vi "Generate Shipping List.vi"(8 "error in (no error)":errorcluster, 10 "Shipping ID":i32, 11 "Delivery in":refnum<class "Delivery.lvclass">) -> (0 "error out":errorcluster, 3 "Delivery out":refnum<class "Delivery.lvclass">)   [LabVIEW 2019, in "Delivery.lvclass"]
uses:
  Delivery.lvclass
  Delivery.lvclass/Delivery.ctl
panel:
  out "Price:":string
  out "Estimated Delivery Time:":string
  out "Transport Company:":string
  out "Parcel Delivery Address":string
  out "Parcel Pickup Address":string
  out "Shipping List ID:":string
  out "Recipient:":string
  in  "Stop":bool
  out "Sender:":string
  # "Shipping List"
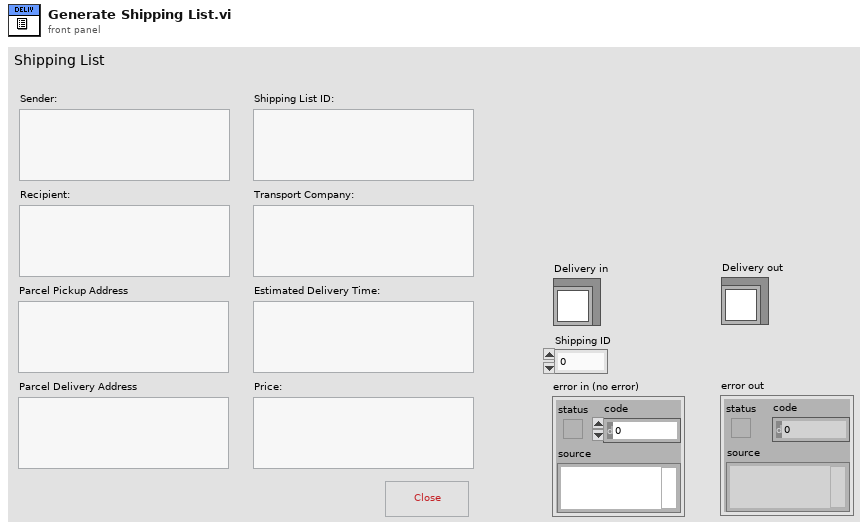
[diagram p1: front panel]
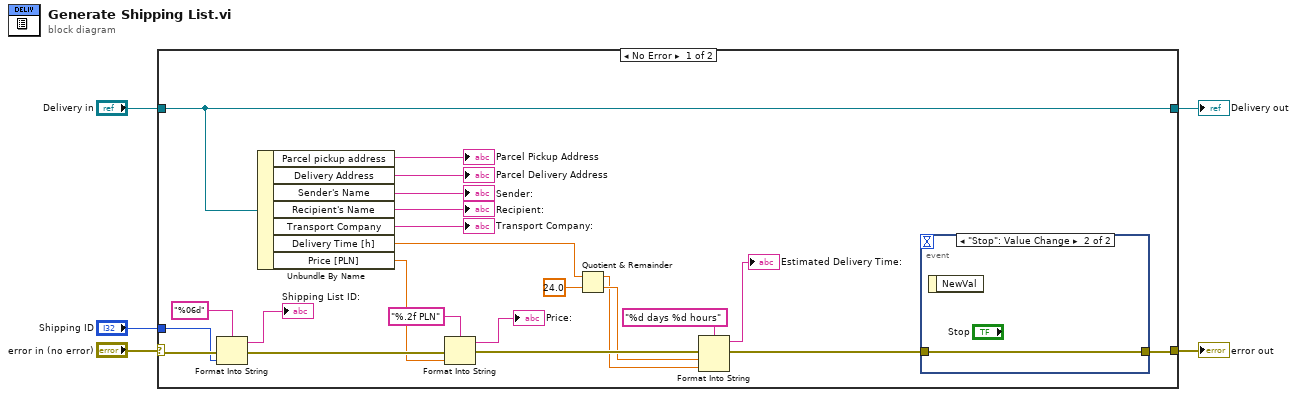
[diagram p0: block diagram]
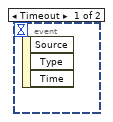
[diagram p2: hidden frame]
diagram:
  n1 = case shown="No Error" "error in (no error)" {
    selector: "error in (no error)" -> [w22 w31]
    tunnel: [w6 w31] -> w4
    tunnel: [w28 w30] -> w2
    tunnel: "Delivery in" -> [w28 w30]
    tunnel: "Shipping ID" -> [w20 _]
    frame No Error {
      n2 = Format Into String(format string="%06d", error in=w22, w20) -> (resulting string=→"Shipping List ID:":string, error out=w18:errorcluster)  [unwired: 1 in]
      n3 = Unbundle By Name(w28) -> ("Parcel pickup address"=→"Parcel Pickup Address":string, "Delivery Address"=→"Parcel Delivery Address":string, "Sender's Name"=→"Sender:":string, "Recipient's Name"=→"Recipient:":string, "Transport Company"=→"Transport Company:":string, "Delivery Time [h]"=w14:dbl, "Price [PLN]"=w17:dbl)
      n4 = Format Into String(format string="%.2f PLN", error in=w18, w17) -> (resulting string=→"Price:":string, error out=w12:errorcluster)  [unwired: 1 in]
      n5 = Quotient & Remainder(x=w14, y=24.0) -> (x-y*floor(x/y)=w9:dbl, floor(x/y)=w10:dbl)
      n6 = Format Into String(format string="%d days %d hours", error in=w12, w10, w9) -> (resulting string=→"Estimated Delivery Time:":string, error out=w7:errorcluster)  [unwired: 1 in]
      n7 = event shown="[1] \"Stop\": Value Change" {
        selector: _ -> [_ _]
        dyn-events: _ -> [_ _]
        timeout: _ -> [_ _]
        tunnel: w7 -> [_ w29]
        tunnel: [_ w29] -> w6
        event Timeout {
          n8 = event-data() -> ()  [unwired: 1 in, 3 out]
        }
        event "Stop": Value Change {
          n9 = event-data() -> ()  [unwired: 1 in, 1 out]
        }
      }
    }
    frame Error {
    }
  }
  "error out" <- w4
  "Delivery out" <- w2
